vi "get tour type.vi"(1 "end square":T1, 2 "start square":T1) -> (0 "tour type":T2)   [LabVIEW 2020, in "core.lvlib"]
uses:
  core.lvlib
  core_data/chessboard_index.ctl
  core_data/tour type (enum).ctl
  core_data/core_data.lvlib
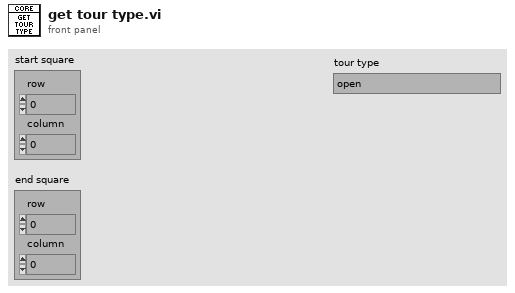
[diagram p1: front panel]
types:
  T1 = typedef "core.lvlib/core_data.lvlib/chessboard_index.ctl" = cluster{"row":u8, "column":u8}
  T2 = typedef "core.lvlib/core_data.lvlib/tour type (enum).ctl" = enum16{"open", "closed"}
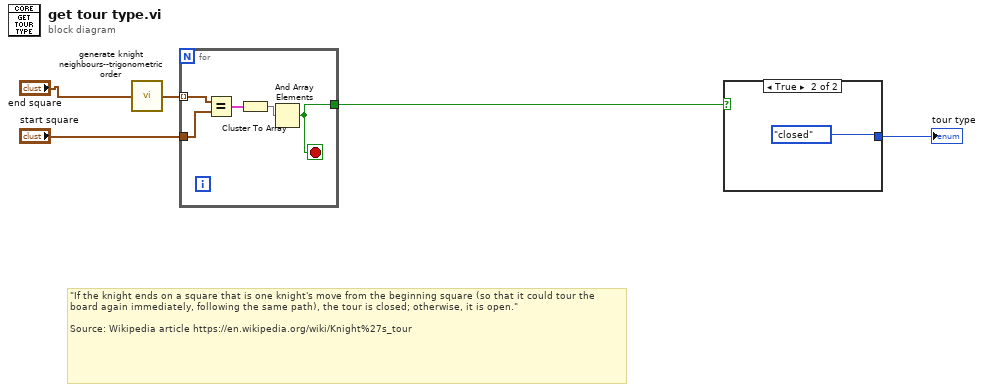
[diagram p0: block diagram]
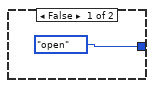
[diagram p2: hidden frame]
diagram:
  # "\"If the knight ends on a square that is one knight's move from the beginning square (so that it could tour the board again immediately, following the same path), the tour is closed; otherwise, it is open.\"\n\nSource: Wikipedia article https://en.wikipedia.org/wiki/Knight%27s_tour"
  n1 = call "generate knight neighbours--trigonometric order.vi"("current square (chessboard_index)"="end square") -> ("neighbours (chessboard_index)"=w4:T1[])
  n2 = for {
    tunnel: w4 -> [w10] mode=indexing
    tunnel: "start square" -> [w9]
    tunnel: [w6] -> w1
    stop <- w6 stop-if-true
    n3 = Equal?(x=w10, y=w9) -> (x = y?=w8:cluster{"row":bool, "column":bool})
    n4 = Cluster To Array(cluster=w8) -> (array=w7:bool[])
    n5 = And Array Elements(Boolean array=w7) -> (logical AND=w6:bool)
  }
  n6 = case shown="True" w1 {
    tunnel: [tour_type_(enum)."open" ("tour type") tour_type_(enum)."closed" ("tour type")] -> w2
    frame False {
    }
    frame True {
    }
  }
  "tour type" <- w2
